vi "Enqueue Last Picture To Undo.vi"(8 "error in (no error)":errorcluster, 9 "Graphics":refnum<class "Graphic.lvclass">[](array[class]), 10 "Last Picture":picture, 11 "Canvas in":refnum<class "Canvas.lvclass">) -> (0 "error out":errorcluster, 3 "Canvas out":refnum<class "Canvas.lvclass">)   [LabVIEW 2015, in "Canvas.lvclass"]
uses:
  Canvas.lvclass
  Graphic/Graphic.lvclass
  Canvas.lvclass/Canvas.ctl
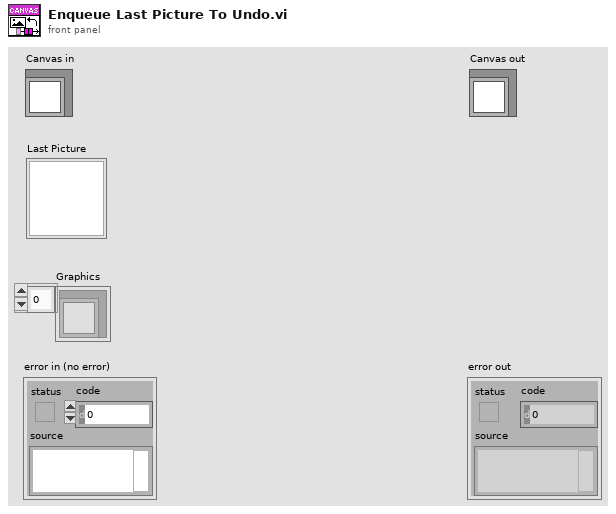
[diagram p1: front panel]
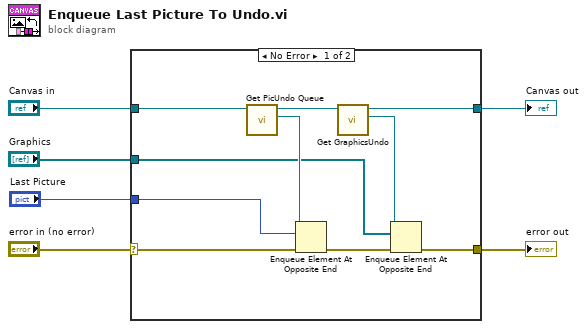
[diagram p0: block diagram]
diagram:
  n1 = case shown="No Error" "error in (no error)" {
    selector: "error in (no error)" -> [w12 w18]
    tunnel: [w7 w18] -> w5
    tunnel: [w11 w17] -> w3
    tunnel: "Canvas in" -> [w16 w17]
    tunnel: "Last Picture" -> [w13 _]
    tunnel: "Graphics" -> [w8 _]
    frame No Error {
      n2 = call "Get PicUndo Queue.vi"("Canvas in"=w16) -> ("Undo Queue"=w14:refnum<queue>, "Canvas out"=w15:refnum<class "Canvas.lvclass">)  [unwired: 8 in, 1 out]
      n3 = Enqueue Element At Opposite End(queue=w14, element=w13, error in (no error)=w12) -> (error out=w9:errorcluster)  [unwired: 1 in, 2 out]
      n4 = call "Get GraphicsUndo.vi"("Canvas in"=w15) -> ("GraphicsUndo"=w10:refnum<queue>, "Canvas out"=w11:refnum<class "Canvas.lvclass">)  [unwired: 8 in, 1 out]
      n5 = Enqueue Element At Opposite End(queue=w10, element=w8, error in (no error)=w9) -> (error out=w7:errorcluster)  [unwired: 1 in, 2 out]
    }
    frame Error {
    }
  }
  "error out" <- w5
  "Canvas out" <- w3
